vi "GetTempsRtd.vi"(5 "error in (no error)":errorcluster) -> (0 "Temp IFD":dbl, 3 "String_Temperatures":string, 4 "Temp RxBox":dbl, 6 "Temp VLNA":dbl, 7 "Temp Outside":dbl, 8 "Temp HLNA":dbl, 9 "Temp ATE Amp":dbl, 10 "Temp H Circ":dbl, 11 "Temp ATE delay":dbl, 12 "Temp V Circ":dbl, 13 "Temp TOF Pwr":dbl, 14 "Temp Siggen":dbl, 15 "Temp Inside":dbl, 16 "Temp V Dummy":dbl, 17 "Temp H Dummy":dbl, 18 "Temp Klystron":dbl, 19 "error out":errorcluster)   [LabVIEW 2009]
doc: "Read multiple temperatures from RTDs"
panel:
  in  "TempSpare2":dbl=-999.0 format="%#.10g"
  in  "TempSpare1":dbl=-999.0 format="%#.10g"
  in  "SCPI command":string="sens:temp:nplc 10,(@1001:1015)\nSENS:TEMP:TRAN:FRTD:RES 100.0,(@1001:1015)\nSENS:TEMP:TRAN:FRTD:TYPE 85,(@1001:1015)\nconf:temp FRTD,85,1,0.001,(@1001:1015)\nrout:scan (@1001:1015)\ninit\n"
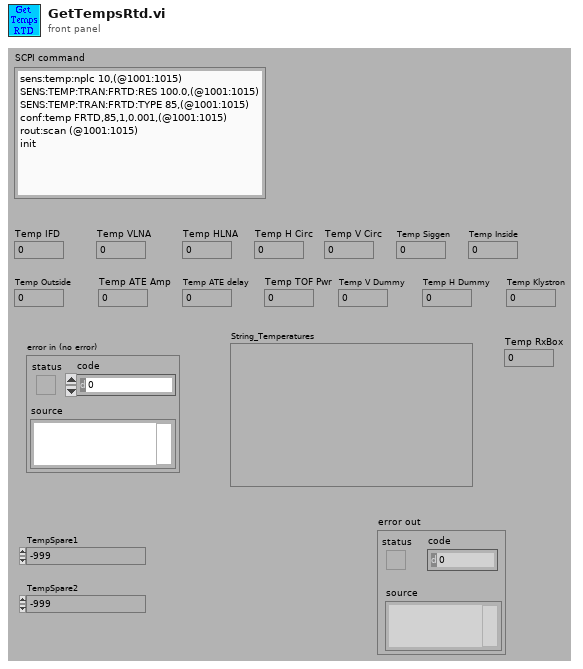
[diagram p1: front panel]
types:
  T1 = enum16{"N1911A", "Siggen", "34980a", "E4418B", "Rvp8"}
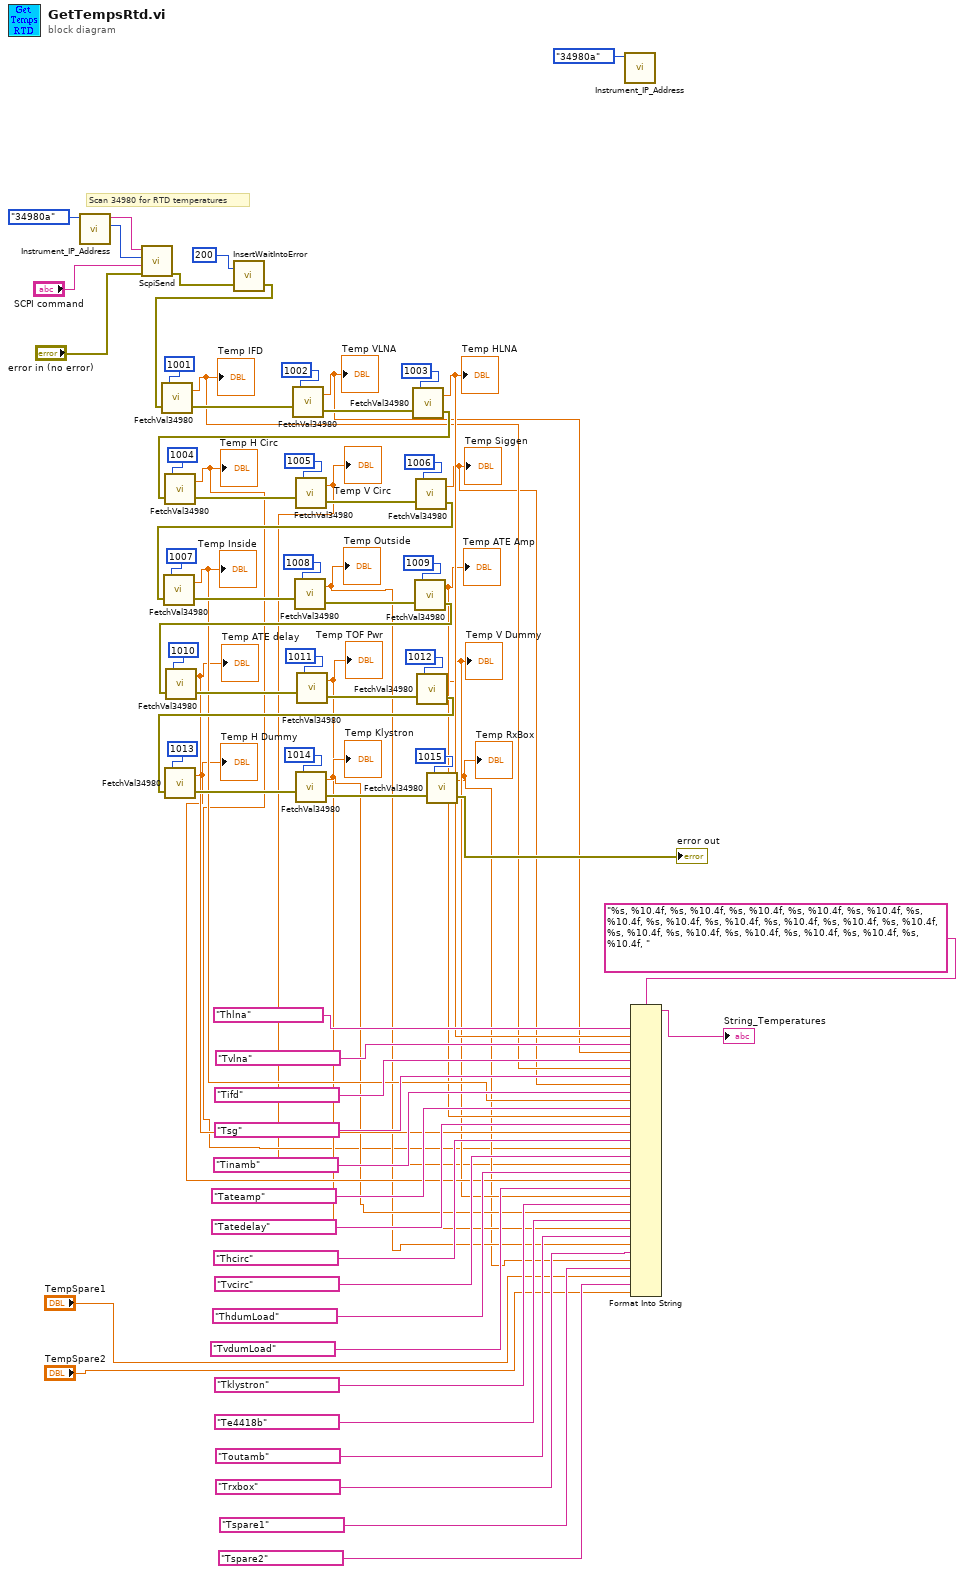
[diagram p0: block diagram]
diagram:
  # "Scan 34980 for RTD temperatures"
  n1 = call "Instrument_IP_Address.vi"("Instrument"=T1."34980a") -> ("Port"=w2:u16, "IP Address"=w3:string)  [unwired: 9 in]
  n2 = call "ScpiSend.vi"("error in (no error)"="error in (no error)", "Command"="SCPI command", "TCP port"=w2, "IP Address"=w3) -> ("error out"=w71:errorcluster)  [unwired: 7 in]
  n3 = call "InsertWaitIntoError.vi"("error in (no error)"=w71, "Wait (msecs)"=200) -> ("error out"=w48:errorcluster)  [unwired: 1 in]
  n4 = call "FetchVal34980.vi"("error in (no error)"=w48, "Circuit ID"=1001) -> ("Error out"=w69:errorcluster, "Value"=w22:dbl)
  "Temp IFD" <- w22
  n5 = call "FetchVal34980.vi"("error in (no error)"=w69, "Circuit ID"=1002) -> ("Error out"=w67:errorcluster, "Value"=w23:dbl)
  "Temp VLNA" <- w23
  n6 = call "FetchVal34980.vi"("error in (no error)"=w67, "Circuit ID"=1003) -> ("Error out"=w47:errorcluster, "Value"=w37:dbl)
  "Temp HLNA" <- w37
  n7 = call "FetchVal34980.vi"("error in (no error)"=w47, "Circuit ID"=1004) -> ("Error out"=w64:errorcluster, "Value"=w11:dbl)
  "Temp H Circ" <- w11
  n8 = call "FetchVal34980.vi"("error in (no error)"=w64, "Circuit ID"=1005) -> ("Error out"=w62:errorcluster, "Value"=w10:dbl)
  "Temp V Circ" <- w10
  n9 = call "FetchVal34980.vi"("error in (no error)"=w62, "Circuit ID"=1006) -> ("Error out"=w46:errorcluster, "Value"=w21:dbl)
  "Temp Siggen" <- w21
  n10 = call "FetchVal34980.vi"("error in (no error)"=w46, "Circuit ID"=1007) -> ("Error out"=w59:errorcluster, "Value"=w20:dbl)
  "Temp Inside" <- w20
  n11 = call "FetchVal34980.vi"("error in (no error)"=w59, "Circuit ID"=1008) -> ("Error out"=w61:errorcluster, "Value"=w13:dbl)
  "Temp Outside" <- w13
  n12 = call "FetchVal34980.vi"("error in (no error)"=w61, "Circuit ID"=1009) -> ("Error out"=w45:errorcluster, "Value"=w19:dbl)
  "Temp ATE Amp" <- w19
  n13 = call "FetchVal34980.vi"("error in (no error)"=w45, "Circuit ID"=1010) -> ("Error out"=w54:errorcluster, "Value"=w18:dbl)
  "Temp ATE delay" <- w18
  n14 = call "FetchVal34980.vi"("error in (no error)"=w54, "Circuit ID"=1011) -> ("Error out"=w52:errorcluster, "Value"=w14:dbl)
  "Temp TOF Pwr" <- w14
  n15 = call "FetchVal34980.vi"("error in (no error)"=w52, "Circuit ID"=1012) -> ("Error out"=w44:errorcluster, "Value"=w16:dbl)
  "Temp V Dummy" <- w16
  n16 = call "FetchVal34980.vi"("error in (no error)"=w44, "Circuit ID"=1013) -> ("Error out"=w51:errorcluster, "Value"=w17:dbl)
  "Temp H Dummy" <- w17
  n17 = call "FetchVal34980.vi"("error in (no error)"=w51, "Circuit ID"=1014) -> ("Error out"=w42:errorcluster, "Value"=w15:dbl)
  "Temp Klystron" <- w15
  n18 = call "FetchVal34980.vi"("error in (no error)"=w42, "Circuit ID"=1015) -> ("Error out"=→"error out":errorcluster, "Value"=w12:dbl)
  "Temp RxBox" <- w12
  n19 = call "Instrument_IP_Address.vi"("Instrument"=T1."34980a") -> ()  [unwired: 9 in, 2 out]
  n20 = Format Into String(format string="%s, %10.4f, %s, %10.4f, %s, %10.4f, %s, %10.4f, %s, %10.4f, %s, %10.4f, %s, %10.4f, %s, %10.4f, %s, %10.4f, %s, %10.4f, %s, %10.4f, %s, %10.4f, %s, %10.4f, %s, %10.4f, %s, %10.4f, %s, %10.4f, %s, %10.4f, ", "Thlna", w37, "Tvlna", w23, "Tifd", w22, "Tsg", w21, "Tinamb", w20, "Tateamp", w19, "Tatedelay", w18, "Thcirc", w11, "Tvcirc", w10, "ThdumLoad", w17, "TvdumLoad", w16, "Tklystron", w15, "Te4418b", w14, "Toutamb", w13, "Trxbox", w12, "Tspare1", "TempSpare1", "Tspare2", "TempSpare2") -> (resulting string=→"String_Temperatures":string)  [unwired: 2 in, 1 out]
